vi "SetVocm.vi"(0 "RIO Device":T1, 1 "ADAPTER NAME":u8(ring) items=["1120 - 1 CH", "1212 - 2 CHs"], 2 "Vocm Offset(V)":dbl, 3 "error in (no error)":errorcluster, 4 "Selected Output":u8(ring) items=["Vout A", "Vout B"]) -> (5 "RIO Device out":T1, 6 "error out":errorcluster)   [LabVIEW 2018]
uses:
  <vilib>/userdefined/High Color/nirio_resource_hc.ctl
  VocmCF_1120.vi
  VocmCF_1212.vi
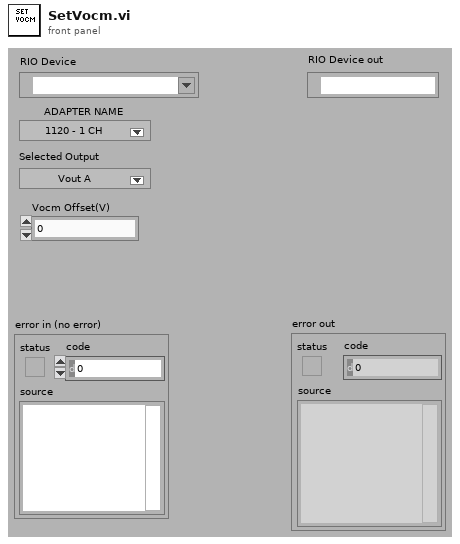
[diagram p1: front panel]
types:
  T1 = typedef "nirio_resource_hc.ctl" = tag
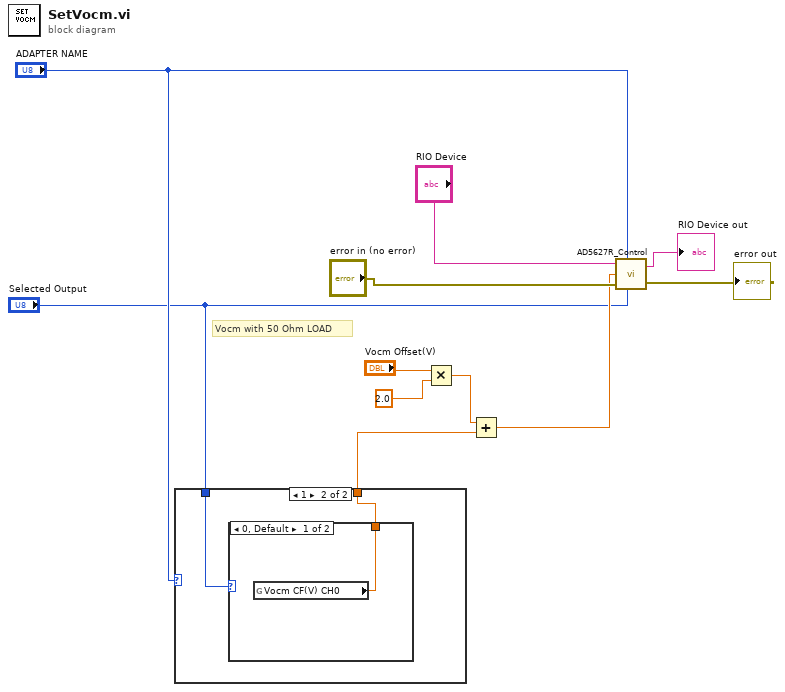
[diagram p0: block diagram]
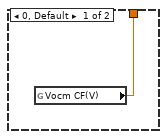
[diagram p2: hidden frame]
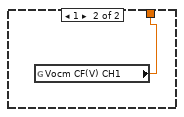
[diagram p3: hidden frame]
diagram:
  # "Vocm with 50 Ohm LOAD"
  n1 = case shown="1" "ADAPTER NAME" {
    tunnel: "Selected Output" -> [_ w14]
    tunnel: [w12 w13] -> w1
    frame 0, Default {
      n2 = global read "VocmCF_1120.vi" "Vocm CF(V)"() -> (w12:dbl)
    }
    frame 1 {
      n3 = case shown="0, Default" w14 {
        tunnel: [w15 w16] -> w13
        frame 0, Default {
          n4 = global read "VocmCF_1212.vi" "Vocm CF(V) CH0"() -> (w15:dbl)
        }
        frame 1 {
          n5 = global read "VocmCF_1212.vi" "Vocm CF(V) CH1"() -> (w16:dbl)
        }
      }
    }
  }
  n6 = Multiply(x="Vocm Offset(V)", y=2.0) -> (x*y=w5:dbl)
  n7 = Add(x=w5, y=w1) -> (x+y=w4:dbl)
  n8 = call "AD5627R_Control.vi"("RIO Device"="RIO Device", "ADAPTER NAME"="ADAPTER NAME", "Vocm Offset(V)"=w4, "error in (no error)"="error in (no error)", "Selected Output"="Selected Output") -> ("RIO Device out"=→"RIO Device out":T1, "error out"=→"error out":errorcluster)
